vi "Get Default Names.vi"(10 "name in":string, 11 "type":T1) -> (2 "name out":string)   [LabVIEW 2021, in "DataTypes_CIF_U.lvlib"]
uses:
  DataTypes_CIF_U.lvlib
  <vilib>/Utility/Data Type/Type Definitions/Data Type.ctl
  <vilib>/Utility/Data Type/NI_Data Type.lvlib
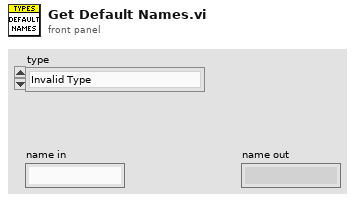
[diagram p1: front panel]
types:
  T1 = typedef "NI_Data Type.lvlib/Data Type.ctl" = enum8{"Invalid Type", "Void", "I8", "I16", "I32", "I64", "U8", "U16", "U32", "U64", "Single Float", "Double Float", "Extended Float", "Single Complex", "Double Complex", "Extended Complex", "Enum U8", "Enum U16", "Enum U32", "Enum U64", "Single Float With Unit", "Double Float With Unit", "Extended Float With Unit", "Single Complex with Unit", "Double Complex with Unit", "Extended Complex with Unit", "Boolean", "String", "Path", "Picture", "Tag", "Array", "Cluster", "Variant", "LV Variant", "Waveform", "Timestamp", "Digital Waveform", "Digital Data", "ExpressData", "Refnum", "External Data", "VI", "Poly VI", "LabVIEW Class Instance", "Fixed Point", "Set Collection", "Map Collection"}
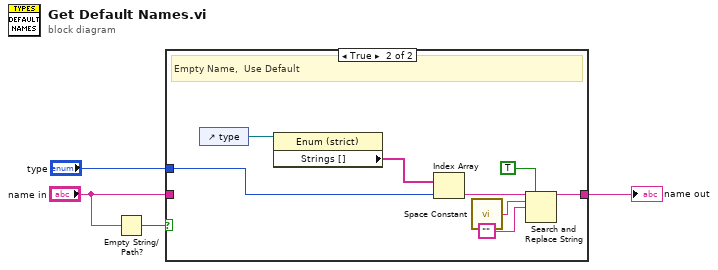
[diagram p0: block diagram]
diagram:
  n1 = Empty String/Path?(string/path="name in") -> (empty?=w4:bool)
  n2 = case shown="True" w4 {
    tunnel: "name in" -> [w5 _]
    tunnel: [w5 w9] -> w2
    tunnel: "type" -> [_ w11]
    frame False {
      # "Valid Name"
    }
    frame True {
      # "Empty Name,  Use Default"
      n3 = control-ref of="type"() -> (w13:refnum<vi>)
      n4 = property class="Enum (strict)"(reference=w13) -> ("Strings []"=w12:string[])  [unwired: 1 in, 2 out]
      n5 = Index Array(array=w12, index=w11) -> (element=w10:string)
      n6 = call <vilib>:"Space Constant.vi"() -> ("String"=w8:string)
      n7 = Search and Replace String(replace all?=TRUE ("replace all? (F)"), input string=w10, search string=w8, replace string="") -> (result string=w9:string)  [unwired: 4 in, 3 out]
    }
  }
  "name out" <- w2
